vi "Configure Sweep Coupling.vi"(0 "VISA resource name":refnum<visa-resource-name>, 1 "Manual VBW/RBW Ratio (1)":dbl=1.0, 2 "Manual Resolution Bandwidth (3E+6 Hz)":i32=3000000 format="%.0g", 3 "Manual Video Bandwidth (3E+6 Hz)":i32=3000001 format="%.0g", 5 "Auto Sweep Time (T: Enable)":bool=TRUE, 7 "Manual Sweep Time (0.0663 s)":dbl=0.0663, 9 "Auto VBW/RBW Ratio (T: Enable)":bool=TRUE, 11 "error in (no error)":errorcluster, 12 "Auto Resolution Bandwidth (T: Enable)":bool=TRUE, 13 "Auto Video Bandwidth (T: Enable)":bool=TRUE) -> (4 "VISA resource name out":refnum<visa-resource-name>, 15 "error out":errorcluster)   [LabVIEW 2014, in "Agilent MXA Series.lvlib"]
doc: "Configures the coupling and sweeping properties of the spectrum analyzer. Resolution bandwidth, video bandwidth, and sweep time can be coupled together by the instrument or set manually.\n\n<B>Note:</B>\nYou can use this VI only under Swept SA, Channel Power Measurement, Occupied Bandwidth, ACP and Burst Power measurement types."
uses:
  Agilent MXA Series.lvlib
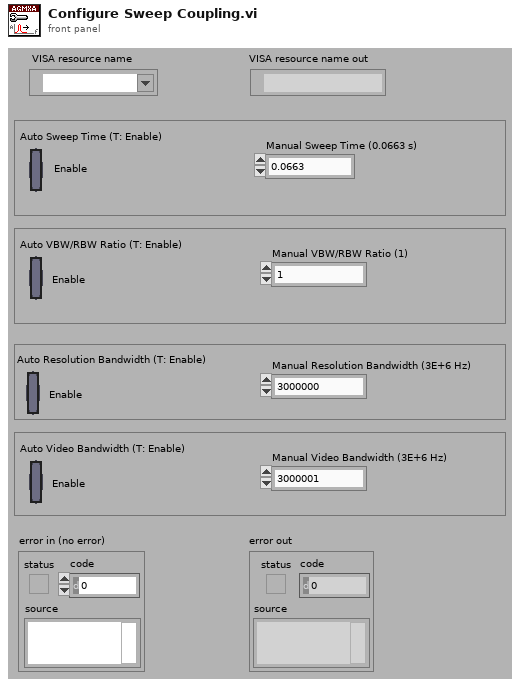
[diagram p1: front panel]
types:
  T1 = typedef "Agilent MXA Series.lvlib/Extended User Data.ctl" = cluster{"Measurement Type":i32, "Agilent MXA/EXA Model":i32}
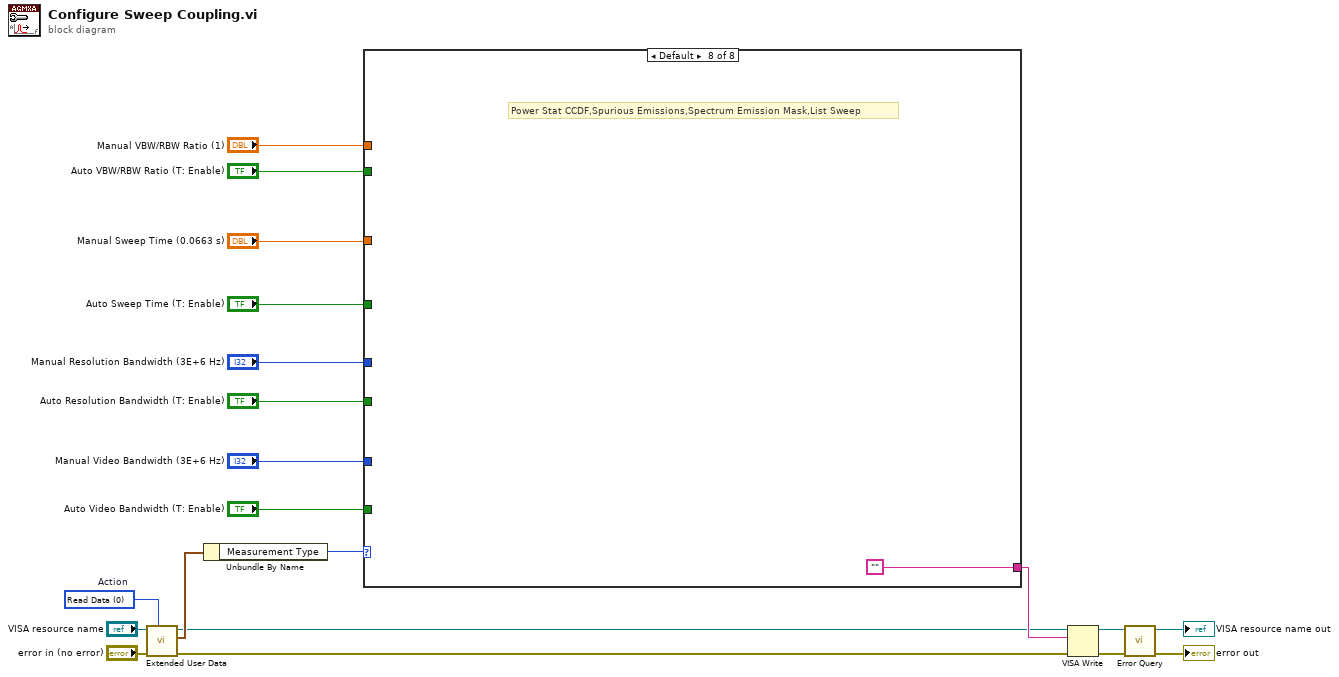
[diagram p0: block diagram]
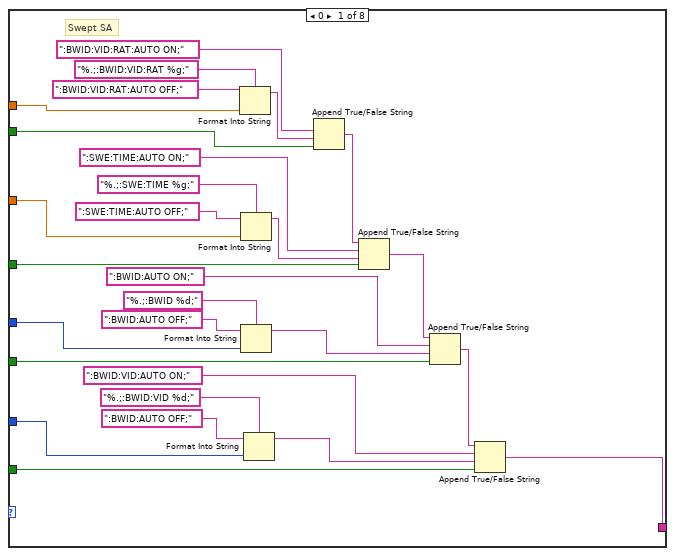
[diagram p2: hidden frame]
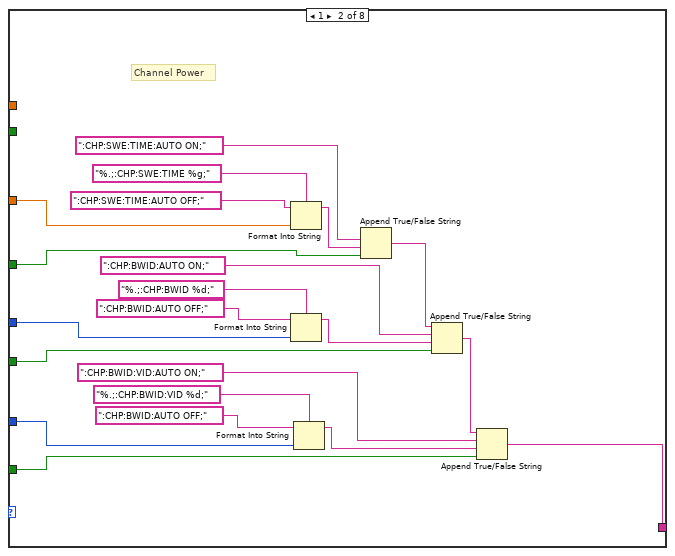
[diagram p3: hidden frame]
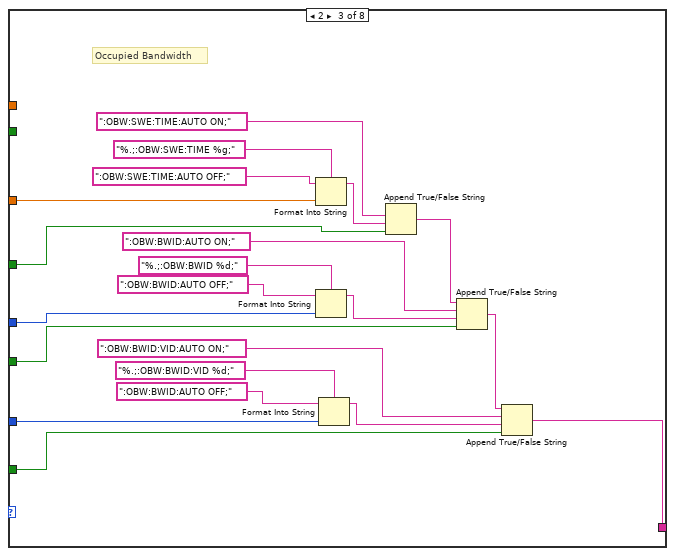
[diagram p4: hidden frame]
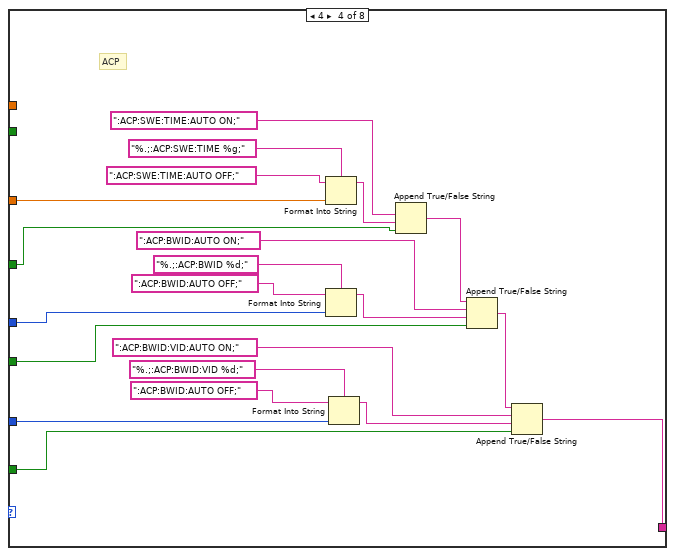
[diagram p5: hidden frame]
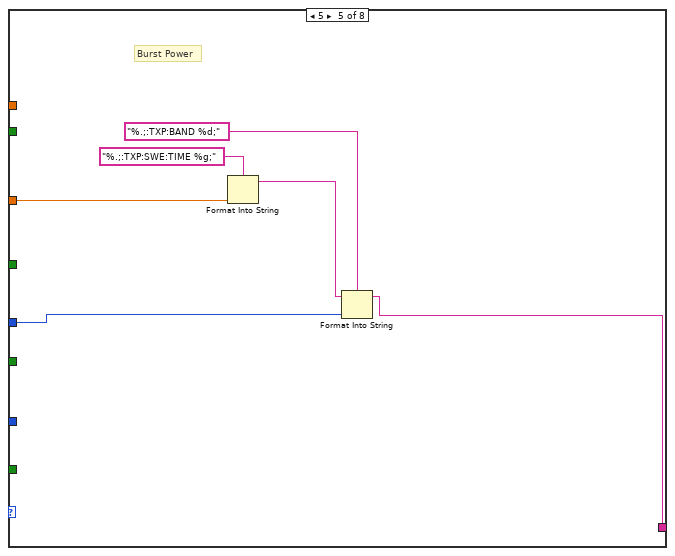
[diagram p6: hidden frame]
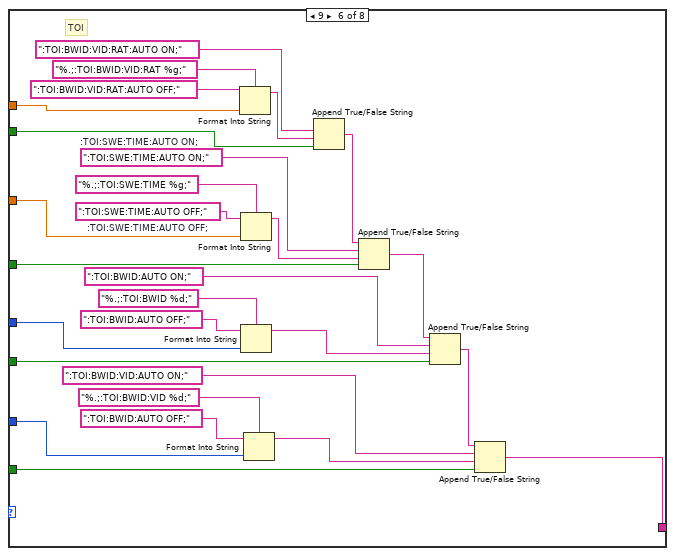
[diagram p7: hidden frame]
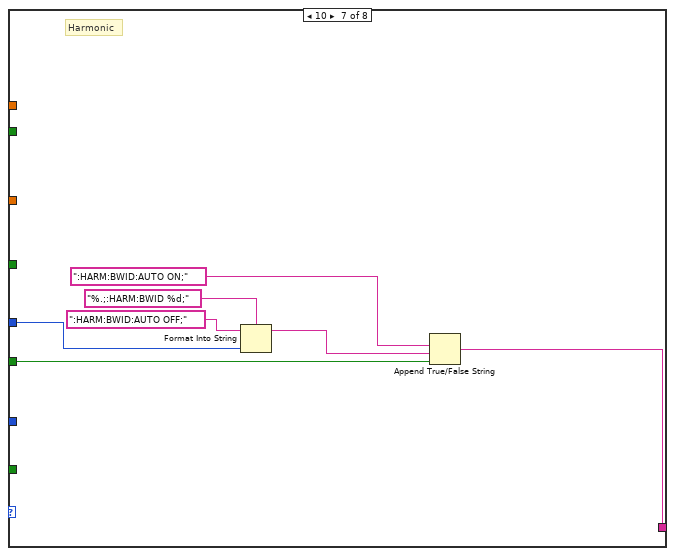
[diagram p8: hidden frame]
diagram:
  w14 = 0 items=["Read Data", "Write Data", "Clear Data", "Clear ALL Data"]  # Action
  n1 = call "Extended User Data.vi"("Action (1:Write Data)"=w14, "Error In (no error)"="error in (no error)", "VISA resource name in"="VISA resource name") -> ("Error Out"=w4:errorcluster, "User Data Out"=w16:T1, "VISA resource name out"=w2:refnum<visa-resource-name>)  [unwired: 6 in]
  n2 = Unbundle By Name(w16) -> ("Measurement Type"=w15:i32)
  n3 = case shown="Default" w15 {
    tunnel: "Auto Sweep Time (T: Enable)" -> [w43 w54 w75 w96 _ w140 _ _]
    tunnel: "Manual Sweep Time (0.0663 s)" -> [w44 w55 w76 w97 w114 w141 _ _]
    tunnel: "Auto VBW/RBW Ratio (T: Enable)" -> [w26 _ _ _ _ w123 _ _]
    tunnel: "Manual Resolution Bandwidth (3E+6 Hz)" -> [w38 w53 w74 w95 w116 w135 w148 _]
    tunnel: "Auto Resolution Bandwidth (T: Enable)" -> [w32 w52 w73 w94 _ w129 w147 _]
    tunnel: "Auto Video Bandwidth (T: Enable)" -> [w30 w50 w71 w92 _ w127 _ _]
    tunnel: "Manual VBW/RBW Ratio (1)" -> [w27 _ _ _ _ w124 _ _]
    tunnel: "Manual Video Bandwidth (3E+6 Hz)" -> [w31 w51 w72 w93 _ w128 _ _]
    tunnel: [w21 w49 w70 w91 w115 w118 w146 ""] -> w5
    frame 0 {
      # "Swept SA"
      n4 = Format Into String(format string="%.;:BWID:VID:RAT %g;", initial string=":BWID:VID:RAT:AUTO OFF;" ("format string"), w27) -> (resulting string=w22:string)  [unwired: 1 in, 1 out]
      n5 = Format Into String(format string="%.;:SWE:TIME %g;", initial string=":SWE:TIME:AUTO OFF;", w44) -> (resulting string=w47:string)  [unwired: 1 in, 1 out]
      n6 = Format Into String(format string="%.;:BWID %d;", initial string=":BWID:AUTO OFF;" ("format string"), w38) -> (resulting string=w39:string)  [unwired: 1 in, 1 out]
      n7 = Format Into String(format string="%.;:BWID:VID %d;", initial string=":BWID:AUTO OFF;" ("format string"), w31) -> (resulting string=w33:string)  [unwired: 1 in, 1 out]
      n8 = Append True/False String(1:w26, 2:w22, 3:":BWID:VID:RAT:AUTO ON;" ("format string")) -> (0:w24:string)  [unwired: 1 in]
      n9 = Append True/False String(1:w43, 2:w47, 3:":SWE:TIME:AUTO ON;", 4:w24) -> (0:w37:string)
      n10 = Append True/False String(1:w32, 2:w39, 3:":BWID:AUTO ON;" ("format string"), 4:w37) -> (0:w25:string)
      n11 = Append True/False String(1:w30, 2:w33, 3:":BWID:VID:AUTO ON;" ("format string"), 4:w25) -> (0:w21:string)
    }
    frame 1 {
      # "Channel Power"
      n12 = Format Into String(format string="%.;:CHP:SWE:TIME %g;", initial string=":CHP:SWE:TIME:AUTO OFF;", w55) -> (resulting string=w68:string)  [unwired: 1 in, 1 out]
      n13 = Format Into String(format string="%.;:CHP:BWID %d;", initial string=":CHP:BWID:AUTO OFF;" ("format string"), w53) -> (resulting string=w62:string)  [unwired: 1 in, 1 out]
      n14 = Format Into String(format string="%.;:CHP:BWID:VID %d;", initial string=":CHP:BWID:AUTO OFF;" ("format string"), w51) -> (resulting string=w57:string)  [unwired: 1 in, 1 out]
      n15 = Append True/False String(1:w54, 2:w68, 3:":CHP:SWE:TIME:AUTO ON;") -> (0:w61:string)  [unwired: 1 in]
      n16 = Append True/False String(1:w52, 2:w62, 3:":CHP:BWID:AUTO ON;" ("format string"), 4:w61) -> (0:w56:string)
      n17 = Append True/False String(1:w50, 2:w57, 3:":CHP:BWID:VID:AUTO ON;" ("format string"), 4:w56) -> (0:w49:string)
    }
    frame 2 {
      # "Occupied Bandwidth"
      n18 = Format Into String(format string="%.;:OBW:SWE:TIME %g;", initial string=":OBW:SWE:TIME:AUTO OFF;", w76) -> (resulting string=w89:string)  [unwired: 1 in, 1 out]
      n19 = Format Into String(format string="%.;:OBW:BWID %d;", initial string=":OBW:BWID:AUTO OFF;" ("format string"), w74) -> (resulting string=w83:string)  [unwired: 1 in, 1 out]
      n20 = Format Into String(format string="%.;:OBW:BWID:VID %d;", initial string=":OBW:BWID:AUTO OFF;" ("format string"), w72) -> (resulting string=w78:string)  [unwired: 1 in, 1 out]
      n21 = Append True/False String(1:w75, 2:w89, 3:":OBW:SWE:TIME:AUTO ON;") -> (0:w82:string)  [unwired: 1 in]
      n22 = Append True/False String(1:w73, 2:w83, 3:":OBW:BWID:AUTO ON;" ("format string"), 4:w82) -> (0:w77:string)
      n23 = Append True/False String(1:w71, 2:w78, 3:":OBW:BWID:VID:AUTO ON;" ("format string"), 4:w77) -> (0:w70:string)
    }
    frame 4 {
      # "ACP"
      n24 = Format Into String(format string="%.;:ACP:SWE:TIME %g;", initial string=":ACP:SWE:TIME:AUTO OFF;", w97) -> (resulting string=w110:string)  [unwired: 1 in, 1 out]
      n25 = Format Into String(format string="%.;:ACP:BWID %d;", initial string=":ACP:BWID:AUTO OFF;" ("format string"), w95) -> (resulting string=w104:string)  [unwired: 1 in, 1 out]
      n26 = Format Into String(format string="%.;:ACP:BWID:VID %d;", initial string=":ACP:BWID:AUTO OFF;" ("format string"), w93) -> (resulting string=w99:string)  [unwired: 1 in, 1 out]
      n27 = Append True/False String(1:w96, 2:w110, 3:":ACP:SWE:TIME:AUTO ON;") -> (0:w103:string)  [unwired: 1 in]
      n28 = Append True/False String(1:w94, 2:w104, 3:":ACP:BWID:AUTO ON;" ("format string"), 4:w103) -> (0:w98:string)
      n29 = Append True/False String(1:w92, 2:w99, 3:":ACP:BWID:VID:AUTO ON;" ("format string"), 4:w98) -> (0:w91:string)
    }
    frame 5 {
      # "Burst Power"
      n30 = Format Into String(format string="%.;:TXP:SWE:TIME %g;", w114) -> (resulting string=w112:string)  [unwired: 2 in, 1 out]
      n31 = Format Into String(format string="%.;:TXP:BAND %d;", initial string=w112, w116) -> (resulting string=w115:string)  [unwired: 1 in, 1 out]
    }
    frame 9 {
      w142 = ":TOI:SWE:TIME:AUTO OFF;"  # :TOI:SWE:TIME:AUTO OFF;
      w143 = ":TOI:SWE:TIME:AUTO ON;"  # :TOI:SWE:TIME:AUTO ON;
      # "TOI"
      n32 = Format Into String(format string="%.;:TOI:BWID:VID:RAT %g;", initial string=":TOI:BWID:VID:RAT:AUTO OFF;" ("format string"), w124) -> (resulting string=w119:string)  [unwired: 1 in, 1 out]
      n33 = Format Into String(format string="%.;:TOI:SWE:TIME %g;", initial string=w142, w141) -> (resulting string=w144:string)  [unwired: 1 in, 1 out]
      n34 = Format Into String(format string="%.;:TOI:BWID %d;", initial string=":TOI:BWID:AUTO OFF;" ("format string"), w135) -> (resulting string=w136:string)  [unwired: 1 in, 1 out]
      n35 = Format Into String(format string="%.;:TOI:BWID:VID %d;", initial string=":TOI:BWID:AUTO OFF;" ("format string"), w128) -> (resulting string=w130:string)  [unwired: 1 in, 1 out]
      n36 = Append True/False String(1:w123, 2:w119, 3:":TOI:BWID:VID:RAT:AUTO ON;" ("format string")) -> (0:w121:string)  [unwired: 1 in]
      n37 = Append True/False String(1:w140, 2:w144, 3:w143, 4:w121) -> (0:w134:string)
      n38 = Append True/False String(1:w129, 2:w136, 3:":TOI:BWID:AUTO ON;" ("format string"), 4:w134) -> (0:w122:string)
      n39 = Append True/False String(1:w127, 2:w130, 3:":TOI:BWID:VID:AUTO ON;" ("format string"), 4:w122) -> (0:w118:string)
    }
    frame 10 {
      # "Harmonic"
      n40 = Format Into String(format string="%.;:HARM:BWID %d;", initial string=":HARM:BWID:AUTO OFF;" ("format string"), w148) -> (resulting string=w149:string)  [unwired: 1 in, 1 out]
      n41 = Append True/False String(1:w147, 2:w149, 3:":HARM:BWID:AUTO ON;" ("format string")) -> (0:w146:string)  [unwired: 1 in]
    }
    frame Default {
      # "Power Stat CCDF,Spurious Emissions,Spectrum Emission Mask,List Sweep"
    }
  }
  n42 = VISA Write(VISA resource name=w2, write buffer=w5, error in (no error)=w4) -> (VISA resource name out=w20:refnum<visa-resource-name>, error out=w18:errorcluster)  [unwired: 1 out]
  n43 = call "Error Query.vi"("error in (no error)"=w18, "VISA resource name"=w20) -> ("error out"=→"error out":errorcluster, "VISA resource name out"=→"VISA resource name out":refnum<visa-resource-name>)  [unwired: 6 in, 2 out]
